vi "puls_width.vi"(1 "Y0":dbl[](array[numeric]), 2 "Y":dbl[](array[numeric]), 3 "X":dbl[](array[numeric])) -> (0 "abs(x)":dbl)   [LabVIEW 2018]
panel:
  out "数值":i32
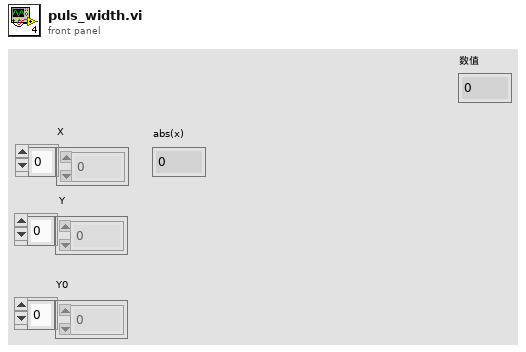
[diagram p1: front panel]
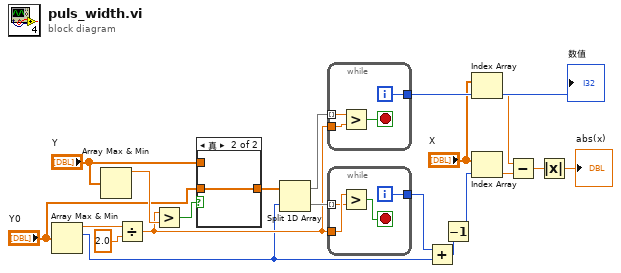
[diagram p0: block diagram]
diagram:
  n1 = Array Max & Min(array="Y0") -> (max value=w20:dbl, max index (indices)=w9:i32)  [unwired: 2 out]
  n2 = Array Max & Min(array="Y") -> (max value=w18:dbl)  [unwired: 3 out]
  n3 = Divide(x=w20, y=2.0) -> (x/y=w11:dbl)
  n4 = Greater?(x=w11, y=w18) -> (0:w17:bool)
  n5 = case shown="真" w17 {
    tunnel: "Y" -> [w21 _]
    tunnel: [w21 w22] -> w15
    tunnel: "Y0" -> [_ w22]
    frame False {
    }
    frame True {
    }
  }
  n6 = Split 1D Array(array=w15, index=w9) -> (first subarray=w13:dbl[], second subarray=w12:dbl[])
  n7 = while {
    tunnel: w13 -> [w26] mode=indexing
    tunnel: w11 -> [w25]
    tunnel: [w23] -> w8
    i -> [w23]
    stop <- w24 stop-if-true
    n8 = Greater?(x=w26, y=w25) -> (0:w24:bool)
  }
  "数值" <- w8
  n9 = while {
    tunnel: w11 -> [w30]
    tunnel: w12 -> [w29] mode=indexing
    tunnel: [w28] -> w10
    i -> [w28]
    stop <- w27 stop-if-true
    n10 = Greater?(x=w30, y=w29) -> (0:w27:bool)
  }
  n11 = Add(x=w10, y=w9) -> (x+y=w6:i32)
  n12 = Decrement(x=w6) -> (x-1=w1:i32)
  n13 = Index Array(array="X", index=w8) -> (element=w5:dbl)
  n14 = Index Array(array="X", index=w1) -> (element=w4:dbl)
  n15 = Subtract(x=w5, y=w4) -> (x-y=w3:dbl)
  n16 = Absolute Value(x=w3) -> (abs(x)=→"abs(x)":dbl)
